vi "Labview_USB_PWM_Test.vi"() -> ()   [LabVIEW 2012]
uses:
  <vilib>/measure/NI_MABase.lvlib
  lib/labview_32bit/ControlPWM/Ginkgo_Driver.dll
panel:
  in  "stops":bool=TRUE
  in  "flag":bool=TRUE
  in  "pInitConfig":T1
  out "error out":errorcluster
  out "Diagram":waveform(dbl)(graph)
  in  "Start":bool
  in  "Stop":bool
  in  "Channel":u16(ring) items=["0", "1", "2", "3", "4", "5", "6", "7"]
  in  "Duty Cycle":u8(slide) scale=0.0..100.0
  in  "Frequency(Hz)":u32(slide) scale=1.0..10000000.0
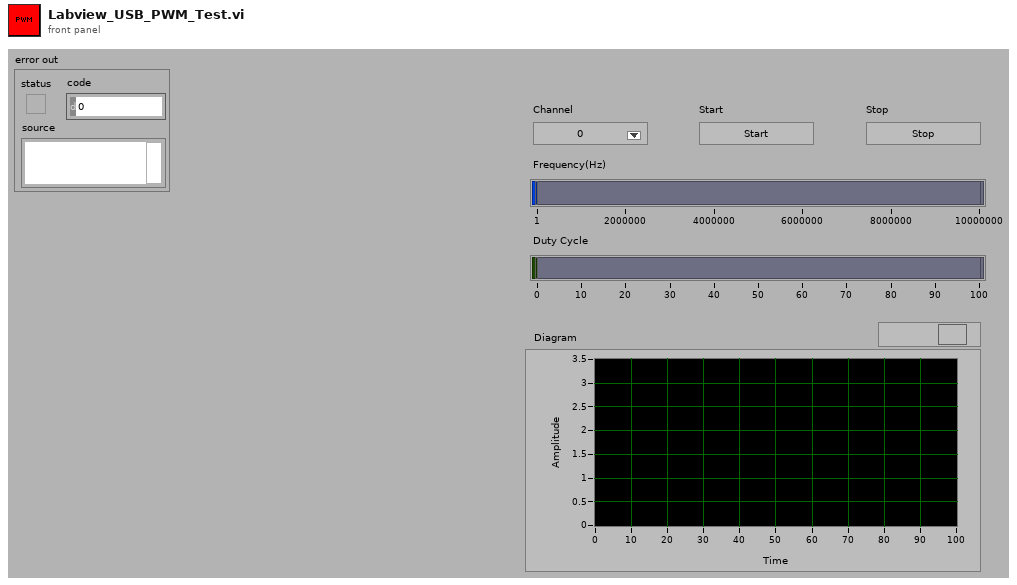
[diagram p1: front panel]
types:
  T1 = cluster{"PWM_ChannelMask":u8, "PWM_Mode":u8, "PWM_Pulse":u8, "PWM_Polarity":u8, "PWM_Frequency":u32}
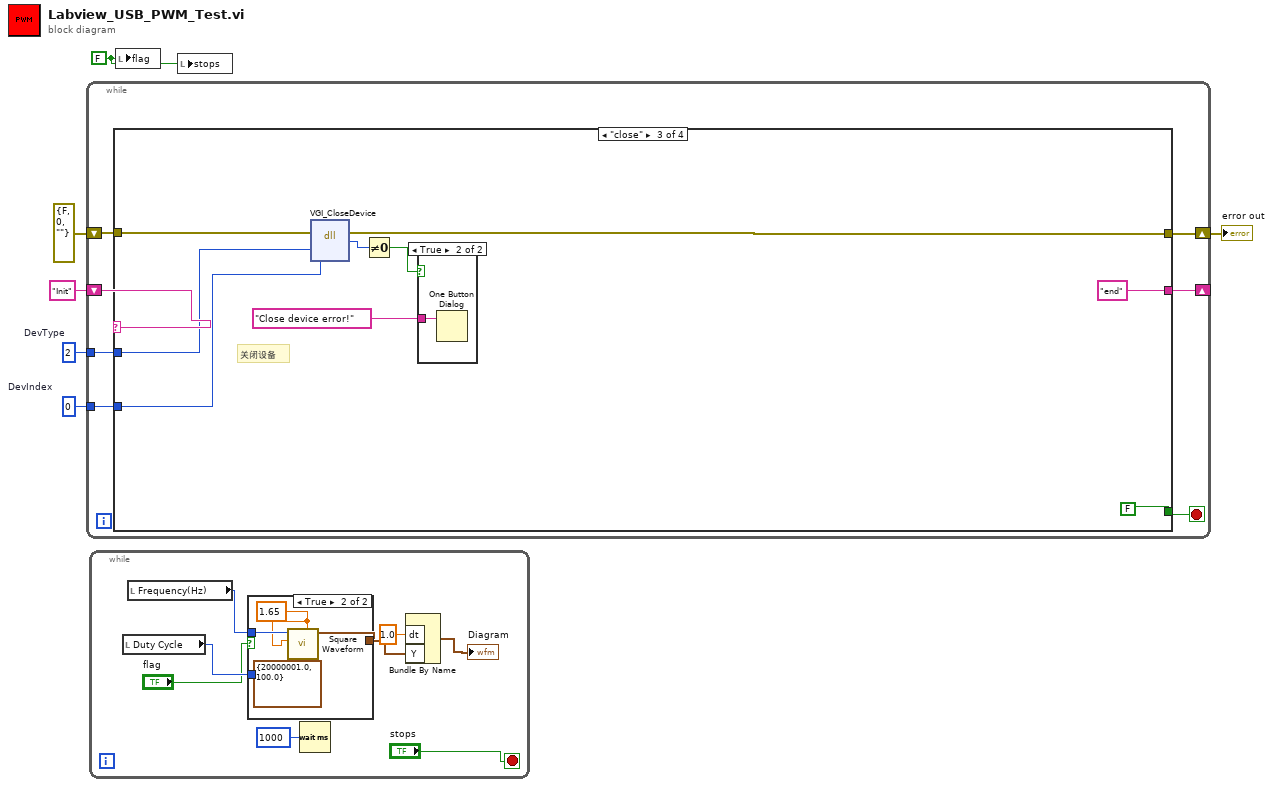
[diagram p0: block diagram]
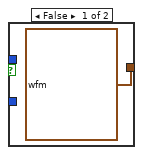
[diagram p2: hidden frame]
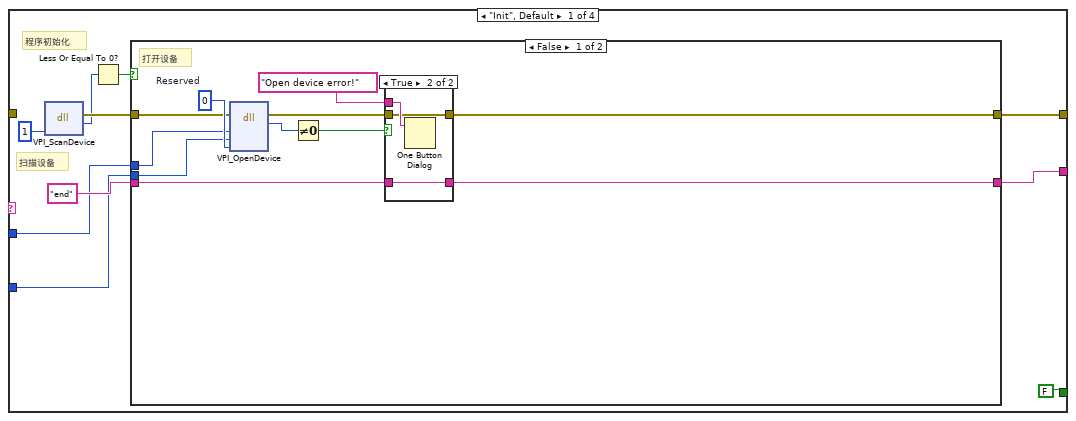
[diagram p3: hidden frame]
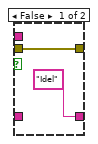
[diagram p4: hidden frame]
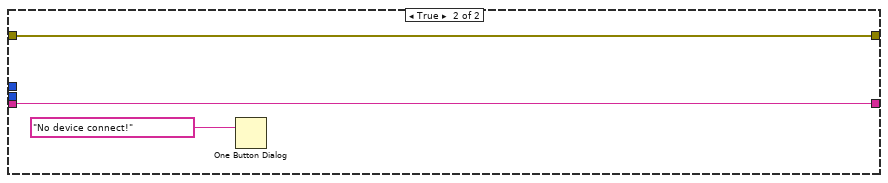
[diagram p5: hidden frame]
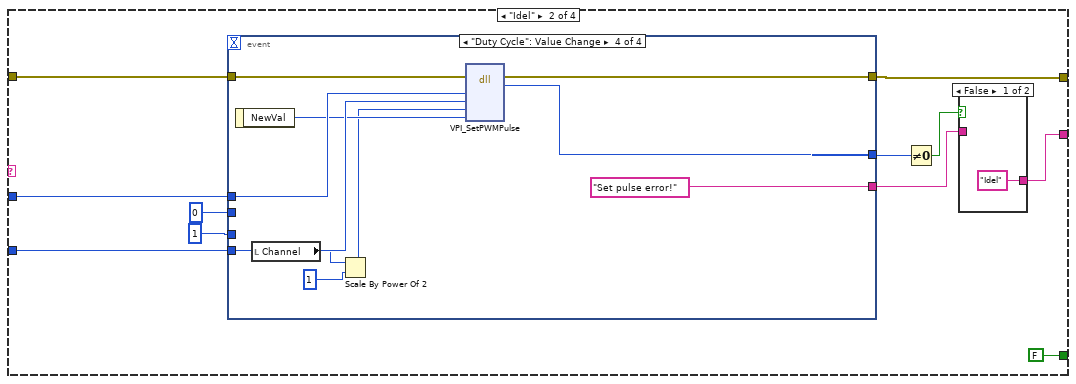
[diagram p6: hidden frame]
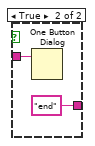
[diagram p7: hidden frame]
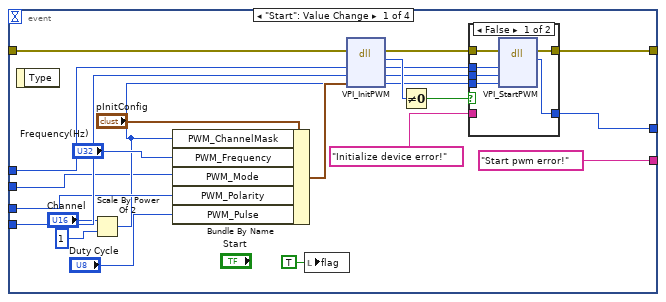
[diagram p8: hidden frame]
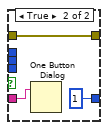
[diagram p9: hidden frame]
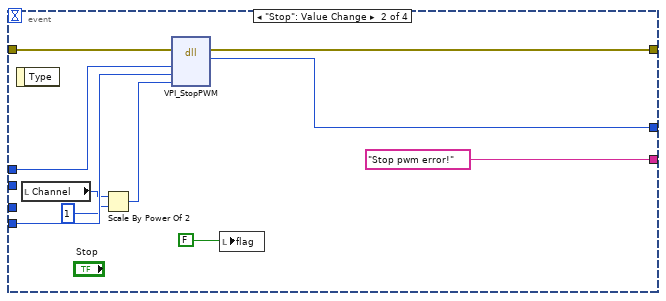
[diagram p10: hidden frame]
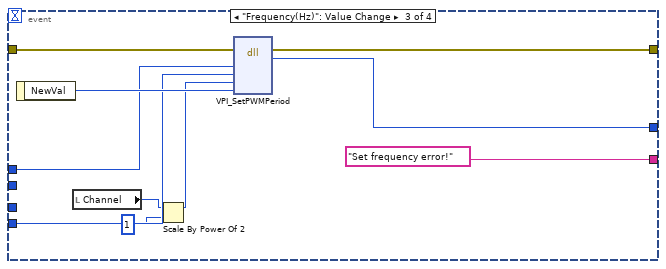
[diagram p11: hidden frame]
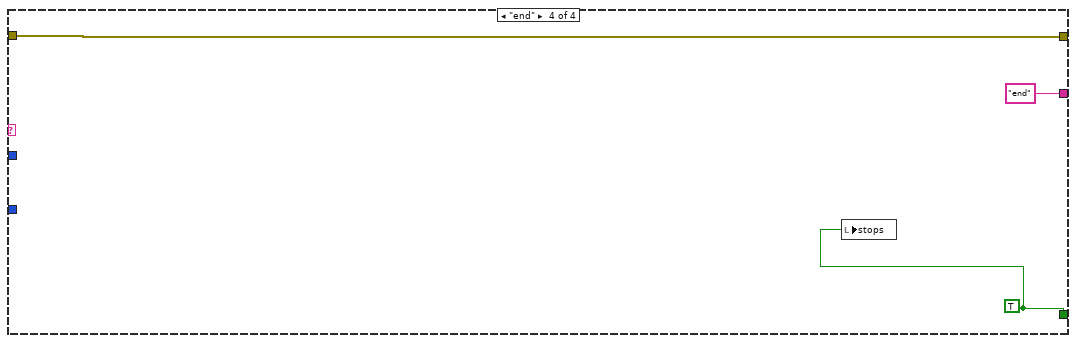
[diagram p13: hidden frame]
diagram:
  w1 = FALSE ("flag")
  w4 = 0  # DevIndex
  w5 = 2  # DevType
  n1 = while {
    shift-right: [w12] -> _
    shift-left: "Init" -> [w13]
    tunnel: w5 -> [w11]
    tunnel: w4 -> [w10]
    shift-right: [w8] -> w3
    shift-left: errorcluster {"status"=FALSE, "code"=0, "source"=""} ("error out") -> [w7]
    stop <- w9 stop-if-true
    n2 = case shown="\"close\"" w13 {
      tunnel: [w18 w45 "end" "end"] -> w12
      tunnel: w11 -> [w17 w52 w117 _]
      tunnel: w10 -> [w16 w51 w118 _]
      tunnel: [FALSE FALSE FALSE w127] -> w9
      tunnel: [w14 w49 w119 w128] -> w8
      tunnel: w7 -> [_ w50 w120 w128]
      frame "Init", Default {
        # "程序初始化"
        # "扫描设备"
        n3 = dll-call lib="E:/Project/vt_ginkgo/truck/Ginkgo Application Example/Labview/Ginkgo PWM/Labview_USB_PWM_Test/lib/labview_32bit/ControlPWM/Ginkgo_Driver.dll" fn="VPI_ScanDevice"("NeedInit"=u8 1) -> (error out=w23:errorcluster, "return type"=w21:i32)  [unwired: 4 in, 1 out]
        n4 = Less Or Equal To 0?(x=w21) -> (x <= 0?=w20:bool)
        n5 = case shown="False" w20 {
          tunnel: w23 -> [w30 w41]
          tunnel: "end" -> [w25 w42]
          tunnel: [w28 w42] -> w18
          tunnel: w17 -> [w24 _]
          tunnel: w16 -> [w27 _]
          tunnel: [w26 w41] -> w14
          frame False {
            w34 = 0  # Reserved
            # "打开设备"
            n6 = dll-call lib="E:/Project/vt_ginkgo/truck/Ginkgo Application Example/Labview/Ginkgo PWM/Labview_USB_PWM_Test/lib/labview_32bit/ControlPWM/Ginkgo_Driver.dll" fn="VPI_OpenDevice"(error in=w30, "DevType"=w24, "DevIndex"=w27, "Reserved"=w34) -> (error out=w29:errorcluster, "return type"=w32:i32)  [unwired: 5 in, 1 out]
            n7 = Not Equal To 0?(x=w32) -> (x != 0?=w31:bool)
            n8 = case shown="True" w31 {
              tunnel: "Open device error!" ("message") -> [_ w39]
              tunnel: w29 -> [w35 w37]
              tunnel: w25 -> [_ w38]
              tunnel: ["Idel" w38] -> w28
              tunnel: [w35 w37] -> w26
              frame False {
              }
              frame True {
                n9 = One Button Dialog(message=w39) -> ()  [unwired: 1 in, 1 out]
              }
            }
          }
          frame True {
            n10 = One Button Dialog(message="No device connect!") -> ()  [unwired: 1 in, 1 out]
          }
        }
      }
      frame "Idel" {
        n11 = event shown="[3] \"Duty Cycle\": Value Change" {
          selector: _ -> [_ _ _ _]
          dyn-events: _ -> [_ _ _ _]
          timeout: _ -> [_ _ _ _]
          tunnel: w52 -> [w75 w96 w105 w116]
          tunnel: w51 -> [w74 w95 w104 w115]
          tunnel: [w64 w93 w102 w112] -> w49
          tunnel: w50 -> [w76 w94 w103 w113]
          tunnel: [w63 w91 w100 w111] -> w48
          tunnel: ["Start pwm error!" "Stop pwm error!" "Set frequency error!" "Set pulse error!"] -> w46
          tunnel: u8 1 ("PWM_Mode") -> [w72 _ _ _]
          tunnel: u8 0 ("PWM_Mode") -> [w57 _ _ _]
          event "Start": Value Change {
            n12 = event-data() -> ()  [unwired: 1 in, 1 out]
            n13 = Scale By Power Of 2(n="Channel", x=u8 1) -> (x*2^n=w58:u8)
            n14 = Bundle By Name(cluster="pInitConfig", "PWM_ChannelMask"=w58, "PWM_Frequency"="Frequency(Hz)", "PWM_Mode"=w57, "PWM_Polarity"=w72, "PWM_Pulse"="Duty Cycle") -> (w71:T1)
            n15 = local write "flag"(TRUE ("flag")) -> ()
            n16 = dll-call lib="E:/Project/vt_ginkgo/truck/Ginkgo Application Example/Labview/Ginkgo PWM/Labview_USB_PWM_Test/lib/labview_32bit/ControlPWM/Ginkgo_Driver.dll" fn="VPI_InitPWM"(error in=w76, "DevType"=w75, "DevIndex"=w74, "pInitConfig"=w71) -> (error out=w67:errorcluster, "return type"=w68:i32, "DevType"=w66:i32, "DevIndex"=w65:i32)  [unwired: 3 in, 1 out]
            n17 = Not Equal To 0?(x=w68) -> (x != 0?=w70:bool)
            n18 = case shown="False" w70 {
              tunnel: "Initialize device error!" -> [_ w87]
              tunnel: w67 -> [w84 w86]
              tunnel: w66 -> [w79 _]
              tunnel: w65 -> [w83 _]
              tunnel: w58 -> [w82 _]
              tunnel: [w81 w86] -> w64
              tunnel: [w80 1] -> w63
              frame False {
                n19 = dll-call lib="E:/Project/vt_ginkgo/truck/Ginkgo Application Example/Labview/Ginkgo PWM/Labview_USB_PWM_Test/lib/labview_32bit/ControlPWM/Ginkgo_Driver.dll" fn="VPI_StartPWM"(error in=w84, "DevType"=w79, "DevIndex"=w83, "ChannelMask"=w82) -> (error out=w81:errorcluster, "return type"=w80:i32)  [unwired: 5 in, 1 out]
              }
              frame True {
                n20 = One Button Dialog(message=w87) -> ()  [unwired: 1 in, 1 out]
              }
            }
          }
          event "Stop": Value Change {
            n21 = event-data() -> ()  [unwired: 1 in, 1 out]
            n22 = local read "Channel"() -> (w89:u16)
            n23 = Scale By Power Of 2(n=w89, x=u8 1) -> (x*2^n=w88:u8)
            n24 = dll-call lib="E:/Project/vt_ginkgo/truck/Ginkgo Application Example/Labview/Ginkgo PWM/Labview_USB_PWM_Test/lib/labview_32bit/ControlPWM/Ginkgo_Driver.dll" fn="VPI_StopPWM"(error in=w94, "DevType"=w96, "DevIndex"=w95, "ChannelMask"=w88) -> (error out=w93:errorcluster, "return type"=w91:i32)  [unwired: 5 in, 1 out]
            n25 = local write "flag"(FALSE ("Boolean")) -> ()
          }
          event "Frequency(Hz)": Value Change {
            n26 = event-data() -> ("NewVal"=w106:u32)  [unwired: 1 in]
            n27 = local read "Channel"() -> (w98:u16)
            n28 = Scale By Power Of 2(n=w98, x=u8 1) -> ()  [unwired: 1 out]
            n29 = dll-call lib="E:/Project/vt_ginkgo/truck/Ginkgo Application Example/Labview/Ginkgo PWM/Labview_USB_PWM_Test/lib/labview_32bit/ControlPWM/Ginkgo_Driver.dll" fn="VPI_SetPWMPeriod"(error in=w103, "DevType"=w105, "DevIndex"=w104, "ChannelMask"=w98, "Frequency"=w106) -> (error out=w102:errorcluster, "return type"=w100:i32)  [unwired: 6 in, 1 out]
          }
          event "Duty Cycle": Value Change {
            n30 = event-data() -> ("NewVal"=w114:u8)  [unwired: 1 in]
            n31 = local read "Channel"() -> (w109:u16)
            n32 = Scale By Power Of 2(n=w109, x=u8 1) -> (x*2^n=w107:u8)
            n33 = dll-call lib="E:/Project/vt_ginkgo/truck/Ginkgo Application Example/Labview/Ginkgo PWM/Labview_USB_PWM_Test/lib/labview_32bit/ControlPWM/Ginkgo_Driver.dll" fn="VPI_SetPWMPulse"(error in=w113, "DevType"=w116, "DevIndex"=w115, "ChannelMask"=w107, "pPulse"=w114) -> (error out=w112:errorcluster, "return type"=w111:i32)  [unwired: 6 in, 1 out]
          }
        }
        n34 = Not Equal To 0?(x=w48) -> (x != 0?=w47:bool)
        n35 = case shown="False" w47 {
          tunnel: w46 -> [_ w56]
          tunnel: ["Idel" "end"] -> w45
          frame False {
          }
          frame True {
            n36 = One Button Dialog(message=w56) -> ()  [unwired: 1 in, 1 out]
          }
        }
      }
      frame "close" {
        # "关闭设备"
        n37 = dll-call lib="E:/Project/vt_ginkgo/truck/Ginkgo Application Example/Labview/Ginkgo PWM/Labview_USB_PWM_Test/lib/labview_32bit/ControlPWM/Ginkgo_Driver.dll" fn="VGI_CloseDevice"(error in=w120, "DevType"=w117, "DevIndex"=w118) -> (error out=w119:errorcluster, "return type"=w123:i32)  [unwired: 4 in, 1 out]
        n38 = Not Equal To 0?(x=w123) -> (x != 0?=w125:bool)
        n39 = case shown="True" w125 {
          tunnel: "Close device error!" ("message") -> [_ w126]
          frame False {
          }
          frame True {
            n40 = One Button Dialog(message=w126) -> ()  [unwired: 1 in, 1 out]
          }
        }
      }
      frame "end" {
        w127 = TRUE
        n41 = local write "stops"(w127) -> ()
      }
    }
  }
  "error out" <- w3
  n42 = while {
    stop <- "stops" stop-if-true
    n43 = local read "Duty Cycle"() -> (w137:u8)
    n44 = local read "Frequency(Hz)"() -> (w136:u32)
    n45 = case shown="True" "flag" {
      tunnel: [waveform(dbl) {"t0"=timestamp(0 s since 1904-01-01), "dt"=1.0, "Y"=[]} ("signal out") w143] -> w134
      tunnel: w137 -> [_ w142]
      tunnel: w136 -> [_ w141]
      frame False {
      }
      frame True {
        w139 = 1.65 ("offset")
        n46 = call <vilib>:"Square Waveform.vi"("duty cycle (%)"=w142, "offset"=w139, "sampling info"=cluster{"Fs":dbl, "#s":dbl} {"Fs"=20000001.0, "#s"=100.0}, "amplitude"=w139, "frequency"=w141) -> ("signal out"=w143:waveform(dbl))  [unwired: 5 in, 1 out]
      }
    }
    n47 = Wait (ms)(milliseconds to wait=u32 1000) -> ()  [unwired: 1 out]
    n48 = Bundle By Name("dt"=1.0, "Y"=w134) -> (→"Diagram":waveform(dbl))  [unwired: 1 in]
  }
  n49 = local write "flag"(w1) -> ()
  n50 = local write "stops"(w1) -> ()
